vi "Window Comparison.vi"() -> ()   [LabVIEW 2009]
doc: "This VI is used to demonstrate the effect of different window functions upon the spectral leakage and low power freqency components of a signal."
uses:
  <vilib>/Analysis/4window.llb/windowTd.ctl
  <vilib>/measure/maspectr.llb/FFT Power Spectrum for N Chan.vi
  <vilib>/measure/NI_MAPro.lvlib
  <vilib>/Analysis/NI_AALPro.lvlib
panel:
  out "Power Spectrum":cluster{"f0":dbl, "df":dbl, "magnitude":dbl[]}[](graph)=[{"f0"=0.0, "df"=1.0, "magnitude"=[-131.32600787836674, -128.30621498094723, -128.27774891797912, -128.23034776893272, -128.16407411852026, -128.0790139108559, -127.97527482224606, -127.85298424516304, -127.71228691707154, -127.55334225946817, -127.37632147517107, -127.18140446625, -126.96877662555208, -126.73862555562023, -126.491137763827, -126.2264953756389, -125.9448728999347, -125.64643407340994, -125.33132880736652, -124.99969024390381, -124.65163192846165, -124.28724509572018, -123.9065960611673, -123.50972370050857, -123.09663700046073, -122.66731265602897, -122.22169267858617, -121.75968199745287, -121.28114599917744, -120.78590797968913, -120.27374645802793, -119.74439230293333, -119.19752562303628, -118.63277235636926, -118.0497004970282, -117.44781588195582, -116.82655745426584, -116.18529190528407, -115.52330758120006, -114.83980752495515, -114.13390149322805, -113.4045967669351, -112.65078752908829, -111.87124254370737, -111.06459080632858, -110.22930476627349, -109.36368062388811, -108.46581508679574, -107.53357781127592, -106.56457855172674, -105.55612777202452, -104.50518911549767, -103.40832165170377, -102.26160916670287, -101.06057286983521, -99.80006264289784, -98.47412019646546, -97.07580496598283, -95.59696987910783, -94.02796860742995, -92.35726750662607, -90.57092232358828, -88.65185869189425, -86.57886059121766, -84.32511119210503, -81.85602371664427, -79.12589958130464, -76.07255264019594, -72.6081876176093, -68.60283491334181, -63.85143704079276, -57.999669112251134, -50.34108702010773, -39.02755314115497, -10.728103632213964, -3.0910408173128117, -7.589836615000372, -35.194072638068405, -48.08108933027512, -56.36640031354936, -62.566215004171724, -67.54152314369541, -71.70388959670495, -75.28491345943758, -78.42867426694316, -81.23120445915787, -83.75984217866221, -86.06368531094346, -88.17966233182466, -90.13626226041809, -91.95593264571244, -93.65667987309348, -95.2531711212648, -96.75751368834169, -98.17981899170569, -99.52861902180817, -100.81117933732713, -102.03373802612336, -103.20169071842426, -104.31973564878659, -105.39198869344865, -106.42207554324796, -107.41320625129448, -108.3682360421081, -109.28971530065716, -110.17993095732811, -111.04094096832901, -111.87460320753333, -112.68259979566588, -113.46645767421862, -114.22756606050918, -114.96719128882904, -115.68648943937097, -116.38651707091795, -117.06824030700378, -117.73254246591026, -118.38023037633205, -119.01203947351496, -119.62863772882619, -120.23062842024233, -120.81855170205742, -121.3928848799743, -121.95404122236232, -122.5023670628633, -123.03813682435843, -123.56154545072997, -124.07269752728574, -124.57159205249526, -125.0581014689785, -125.53194290497352, -125.99263878011746, -126.43946266593582, -126.87136444866285, -127.28686612732895, -127.68391545231535, -128.0596784365957, -128.41024242837912, -128.73018747047226, -129.01196320703662, -129.24498002584176, -129.41428718802794, -129.4986766383771, -129.46805072007896, -129.28000466768492, -128.87594861902963, -128.17787387982554, -127.087815823366, -125.49181184392913, -123.26630836069404, -120.27742361718025, -116.35721604798553, -111.23607110061246, -104.37601361338942, -94.42655516071382, -75.28646117979386, -63.785483979326365, -65.29169056572441, -82.33988715317165, -97.6032381781905, -106.78118473931774, -113.57606421566183, -119.0774519288062, -123.7765675374351, -127.9321818597393, -131.67757872430357, -135.04953628406105, -137.98870626905367, -140.3571802275503, -142.03160052909726, -143.03596395412578, -143.54939208798268, -143.78184233192187, -143.88423545534135, -143.9408028151458, -143.9921016604115, -144.05540002940123, -144.13669072445254, -144.23684145674963, -144.3545642154017, -144.4878040551757, -144.63436728270545, -144.79218861249774, -144.95942907496044, -145.13449651586737, -145.31603263944592, -145.5028874230249, -145.69409059901287, -145.88882447431527, -146.08639968775947, -146.2862343558215, -146.48783648809442, -146.69078925970342, -146.89473881335732, -147.099384111054, -147.30446855844667, -147.5097730442294, -147.71511015360724, -147.92031936741677, -148.1252630445945, -148.32982305556106, -148.53389797764243, -148.73740070428622, -148.9402564490353, -149.14240104911, -149.3437795158948, -149.54434480641834, -149.74405678817, -149.9428813116919, -150.14078946756072, -150.33775690221955, -150.53376324851132, -150.7287916255743, -150.92282821422162, -151.11586187581742, -151.3078838267952, -151.4988873500546, -151.6888675685212, -151.87782117724186, -152.06574630142515, -152.25264230085526, -152.4385096316488, -152.62334969957942, -152.80716477610866, -152.98995784903718, -153.17173256996466, -153.35249317155592, -153.53224438929854, -153.71099135269202, -153.88873960582373, -154.0654950143637, -154.24126372428947, -154.41605212747953, -154.589866819388, -154.76271456917334, -154.93460230727618, -155.10553705870421, -155.27552596483284, -155.44457624364486, -155.6126951697921, -155.77989006139867, -155.94616825735895, -156.11153712855045, -156.27600402689131, -156.43957631648397, -156.60226133519058, -156.7640663929604, -156.92499878472788, -157.0850657320586, -157.24427445798767, -157.4026320933982, -157.56014573606546, -157.716822427362, -157.87266912468192, -158.0276927474128, -158.18190012019676, -158.33529801676985, -158.48789312299343, -158.63969207480605, -158.79070138984576, -158.940927540481, -159.09037690456276, -159.2390557953837, -159.38697042500368, -159.53412694509416, -159.68053140210168, -159.82618979193234, -159.9711079868126, -160.11529181918078, -160.25874700211045, -160.40147919323516, -160.54349395010266, -160.68479676715214, -160.82539302459597, -160.9652880656063, -161.10448710526896, -161.24299527106783, -161.38081777323754, -161.51795946019087, -161.65442530506465, -161.7902201544642, -161.92534874398865, -162.05981577494012, -162.19362584818737, -162.32678348147044, -162.45929314331187, -162.5911591896043, -162.7223859307357, -162.85297761454333, -162.98293835188176, -163.11227226018784, -163.2409833264643, -163.36907548267249, -163.49655260955052, -163.62341848170138, -163.74967684133549, -163.87533131881014, -164.0003855173776, -164.12484294436294, -164.24870705028235, -164.37198120551628, -164.49466873413604, -164.6167728811115, -164.7382968176555, -164.8592436753276, -164.97961647784797, -165.0994182533504, -165.21865187851972, -165.3373202446818, -165.45542614189756, -165.57297228298637, -165.68996135509323, -165.8063959754928, -165.9222786596862, -166.03761193508456, -166.1523982064083, -166.26663983490116, -166.38033913988633, -166.49349834107838, -166.60611966804456, -166.71820520724162, -166.82975705645433, -166.94077723765886, -167.05126764660508, -167.16123023750313, -167.27066686701264, -167.37957921947103, -167.4879690860123, -167.59583810480729, -167.70318792875224, -167.81002006909398, -167.9163360649382, -168.0221373318169, -168.12742524341505, -168.23220115926705, -168.33646634322292, -168.4402220290035, -168.54346928929573, -168.64620938009006, -168.74844325710356, -168.8501719545144, -168.9513964030981, -169.05211749779954, -169.15233607632956, -169.25205290892796, -169.35126871981782, -169.44998423818913, -169.5481999644309, -169.64591658221596, -169.7431345374362, -169.83985429455058, -169.93607625184794, -170.03180075157945, -170.12702811238543, -170.22175854993858, -170.31599223304204, -170.4097293169604, -170.50296987535748, -170.595713931081, -170.68796142715098, -170.7797122805951, -170.87096640035696, -170.9617235175465, -171.05198344655196, -171.1417458374456, -171.2310103313892, -171.31977658059125, -171.40804401820245, -171.49581217977928, -171.58308049445137, -171.6698483297596, -171.75611496938404, -171.84187969955985, -171.92714175717703, -172.01190020091474, -172.09615422255058, -172.17990275440377, -172.26314512723218, -172.34587968067612, -172.42810575647417, -172.50982201679466, -172.59102728681393, -172.67172023923789, -172.75189955450853, -172.83156382865113, -172.91071168142787, -172.98934151111501, -173.06745177223607, -173.14504090023902, -173.2221072419749, -173.29864908739324, -173.37466457614343, -173.4501520457153, -173.52510945871015, -173.59953498957165, -173.6734266099737, -173.7467823226329, -173.81959997752617, -173.89187752810048, -173.963612712844, -174.0348033350739, -174.1054470441478, -174.1755415716635, -174.24508451415718, -174.31407334127755, -174.3825057044271, -174.45037891170105, -174.51769053973635, -174.58443785155936, -174.65061818862546, -174.71622879549165, -174.78126691884867, -174.84572981034614, -174.90961441531442, -174.9729180835028, -175.03563765313604, -175.09777017352184, -175.15931275938607, -175.22026223776166, -175.2806153547823, -175.340369262681, -175.39952040605817, -175.4580659308601, -175.5160023887115, -175.57332644156708, -175.630035104731, -175.68612448650327, -175.74159079512899, -175.79643250778594, -175.8506443956498, -175.90422360382797, -175.95716633667712, -176.00946970773802, -176.0611295708303, -176.11214263367958, -176.1625052976386, -176.21221381200598, -176.26126491169975, -176.3096547753054, -176.35737963989908, -176.40443605830933, -176.45082027193243, -176.49652869590213, -176.54155764601109, -176.5859034130003, -176.62956248353316, -176.67253093364192, -176.71480545703326, -176.75638215128652, -176.79725743682056, -176.83742778109865, -176.87688945046864, -176.915638891146, -176.953672589257, -176.99098691080977, -177.0275783338677, -177.06344341079142, -177.098578515221, -177.13298036448288, -177.1666454878013, -177.19957042364652, -177.2317519121395, -177.26318666000725, -177.29387131699465, -177.32380269991236, -177.35297766658812, -177.38139319593392, -177.4090458767518, -177.43593301409646, -177.46205154916294, -177.48739855695607, -177.51197125563493, -177.53576682043473, -177.5587825380364, -177.58101577470785, -177.60246405565013, -177.62312495121037, -177.64299534114457, -177.6620738011748, -177.6803576096973, -177.69784467270546, -177.71453286729297, -177.7304201935574, -177.74550467074843, -177.7597844801478, -177.77325796633986, -177.78592327280464, -177.797778902976, -177.808823470704, -177.81905551771584, -177.82847376169227, -177.83707705233283, -177.8448642794966, -177.85183445511967, -177.85798670763413, -177.863320191701, -177.86783434748966, -177.87152854820545, -177.87440228634517, -177.87645525615744, -177.87768712336958]}]
  in  "Frequency 2":dbl(knob)=75.12 scale=0.0..200.0
  in  "Frequency 1":dbl(knob)=155.37 scale=0.0..200.0
  in  "Amplitude 2":dbl=1.0
  in  "Amplitude 1":dbl=0.001
  in  "stop":bool
  out "Sine1 + Sine2":dynamicdata(graph)=[{"t0"=timestamp(2181 s since 1904-01-01), "dt"=0.001, "Y"=array[1000 elements], "attributes"=variant("NI_ChannelName"=variant(string "Sine1"), "NI_ExpIsRelativeTime"=variant(bool TRUE), "NI_ExpStartTimeStamp"=variant(timestamp timestamp(3346093281.921332 s since 1904-01-01)), "NI_ExpTimeStamp"=variant(timestamp timestamp(3346095462.921332 s since 1904-01-01)), "NI_ExpXDimension"=variant(string "t"))}]
  in  "window":T1=1 items=["Rectangle"=0, "Hanning"=1, "Hamming"=2, "Blackman-Harris"=3, "Exact Blackman"=4, "Blackman"=5, "Flat Top"=6, "4 Term B-Harris "=7, "7 Term B-Harris"=8, "Low Sidelobe"=9, "Blackman Nuttall"=11, "Triangle"=30, "Bartlett-Hanning"=31, "Bohman"=32, "Parzen"=33, "Welch"=34, "Kaiser"=60, "Dolph-Chebyshev"=61, "Gaussian"=62]
  # "Sine Wave 1"
  # "Sine Wave 2"
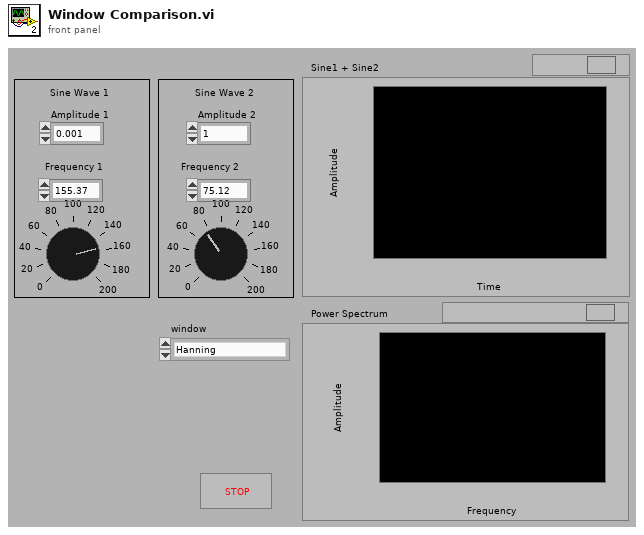
[diagram p1: front panel]
types:
  T1 = typedef "NI_AALPro.lvlib/windowTd.ctl" = u32
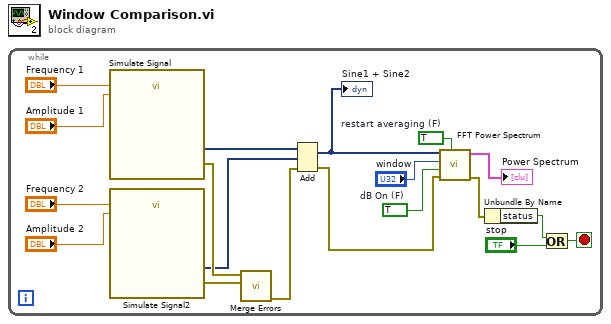
[diagram p0: block diagram]
diagram:
  n1 = while {
    stop <- w10 stop-if-true
    w17 = TRUE  # restart averaging (F)
    w18 = TRUE  # dB On (F)
    n2 = call "Simulate Signal"("Frequency"="Frequency 1", "Amplitude"="Amplitude 1") -> ("Sine1"=w16:dynamicdata, "error out"=w14:errorcluster)  [unwired: 12 in]
    n3 = call "Simulate Signal2"("Frequency"="Frequency 2", "Amplitude"="Amplitude 2") -> ("Sine2"=w1:dynamicdata, "error out"=w4:errorcluster)  [unwired: 12 in]
    n4 = call <vilib>:"Merge Errors.vi"("error in 2 (no error)"=w4, "error in 1 (no error)"=w14) -> ("error out"=w3:errorcluster)  [unwired: 5 in]
    n5 = Add(1:w1, 2:w16, 4:w3) -> (0:w15:dynamicdata, 3:w2:errorcluster)
    "Sine1 + Sine2" <- w15
    n6 = call-poly <vilib>:"FFT Power Spectrum.vi"("restart averaging (F)"=w17, "error in (no error)"=w2, "dB On (F)"=w18, "window"="window", "time signals"=w15) -> ("error out"=w13:errorcluster, "power spectra"=→"Power Spectrum":cluster{"f0":dbl, "df":dbl, "magnitude":dbl[]}[])  [unwired: 3 in, 2 out]
    n7 = Unbundle By Name "Unbundle By Name"(w13) -> ("status"=w12:bool)
    n8 = Or(x=w12, y="stop") -> (x .or. y?=w10:bool)
  }
